vi "ClientTake2.vi"() -> ()   [LabVIEW 2021]
panel:
  in  "stop":bool
  in  "C6":bool
  in  "C5":bool
  in  "C4":bool
  in  "C3":bool
  in  "C2":bool
  in  "C1":bool
  in  "B6":bool
  in  "B5":bool
  in  "B4":bool
  in  "B3":bool
  in  "B2":bool
  in  "B1":bool
  in  "A6":bool
  in  "A5":bool
  in  "A4":bool
  in  "A3":bool
  in  "A2":bool
  in  "A1":bool
  # "1"
  # "2"
  # "3"
  # "4"
  # "5"
  # "6"
  # "Alarm Switches"
  # "Zone"
  # "Bypass Switches"
  # "Tamper Switches"
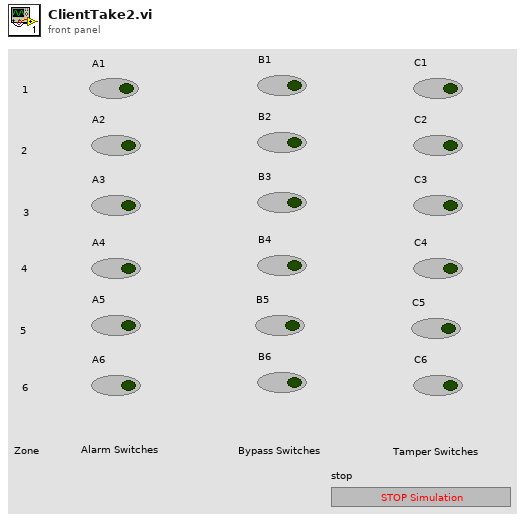
[diagram p1: front panel]
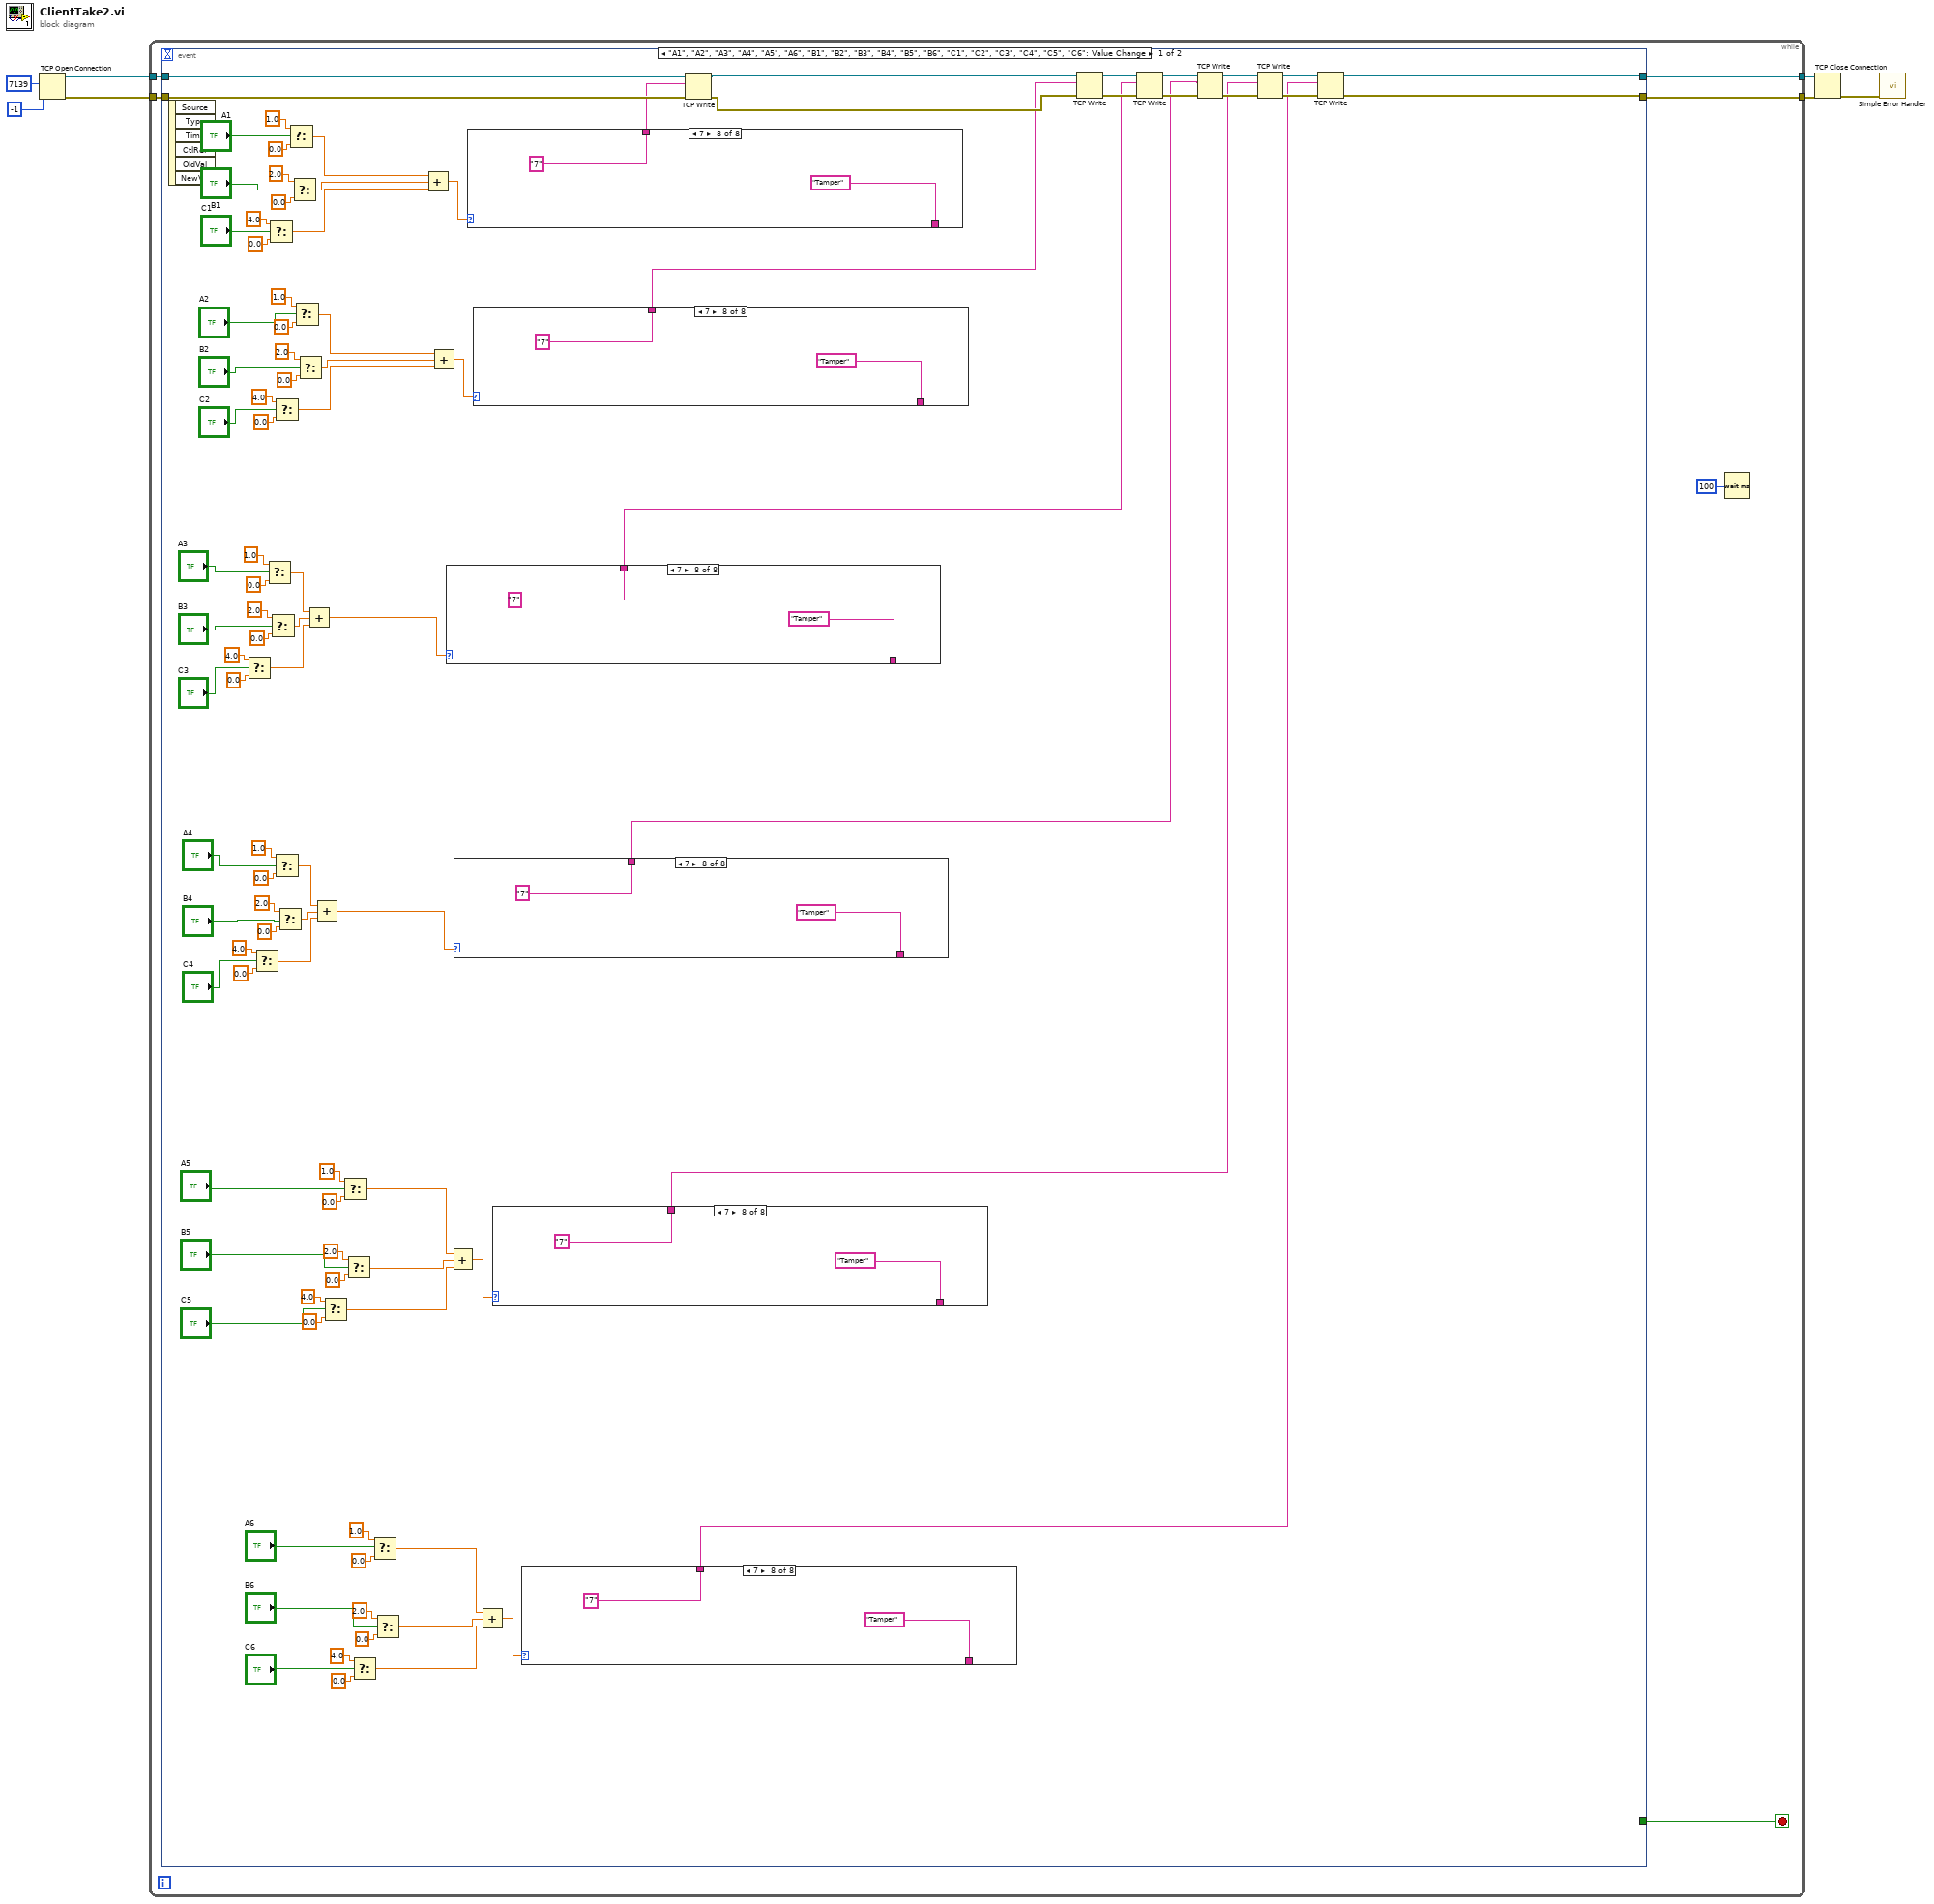
[diagram p0: block diagram]
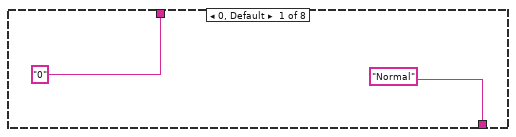
[diagram p2: hidden frame]
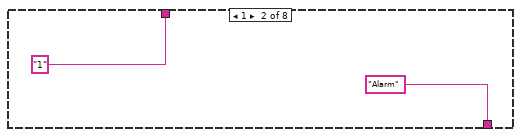
[diagram p3: hidden frame]
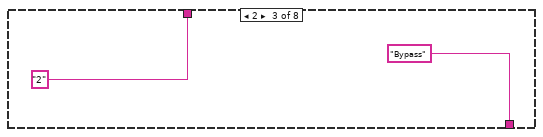
[diagram p4: hidden frame]
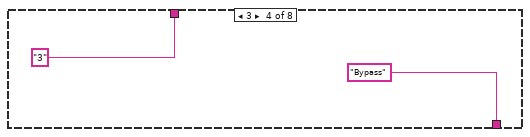
[diagram p5: hidden frame]
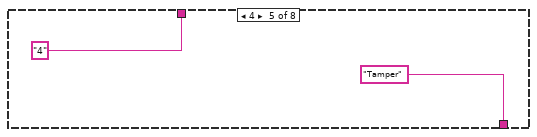
[diagram p6: hidden frame]
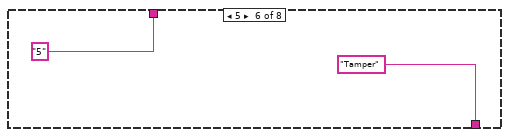
[diagram p7: hidden frame]
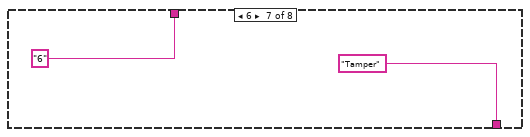
[diagram p8: hidden frame]
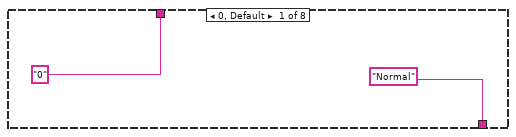
[diagram p9: hidden frame]
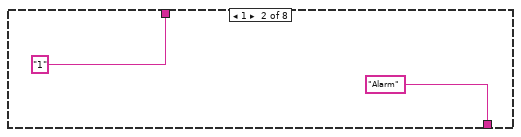
[diagram p10: hidden frame]
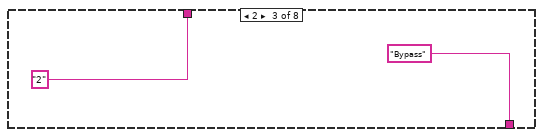
[diagram p11: hidden frame]
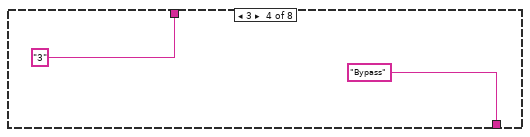
[diagram p12: hidden frame]
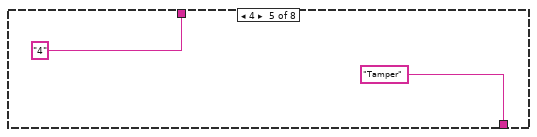
[diagram p13: hidden frame]
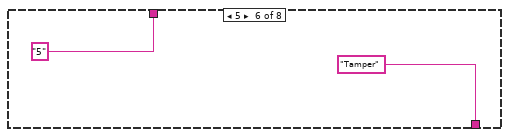
[diagram p14: hidden frame]
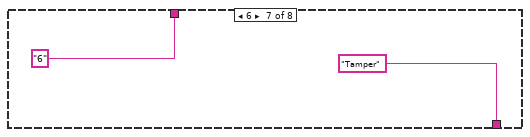
[diagram p15: hidden frame]
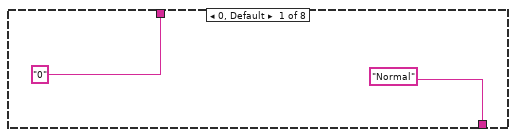
[diagram p16: hidden frame]
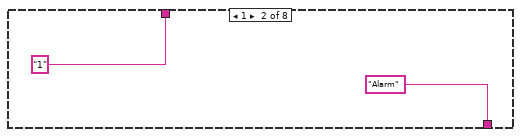
[diagram p17: hidden frame]
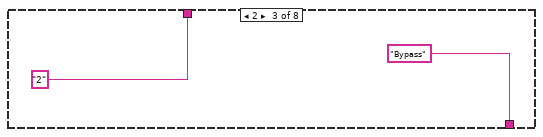
[diagram p18: hidden frame]
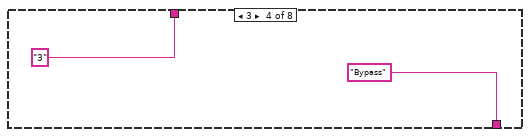
[diagram p19: hidden frame]
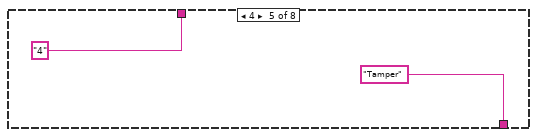
[diagram p20: hidden frame]
diagram:
  n1 = TCP Open Connection(remote port or service name=u16 7139, timeout ms (60000)=-1) -> (connection ID=w7:refnum<k5>, error out=w5:errorcluster)  [unwired: 3 in]
  n2 = while {
    tunnel: w7 -> [w13]
    tunnel: [w10] -> w6
    tunnel: w5 -> [w12]
    tunnel: [w9] -> w4
    stop <- w8 stop-if-true
    n3 = event shown="[0] \"A1\", \"A2\", \"A3\", \"A4\", \"A5\", \"A6\", \"B1\", \"B2\", \"B3\", \"B4\", \"B5\", \"B6\", \"C1\", \"C2\", \"C3\", \"C4\", \"C5\", \"C6\": Value Change" {
      selector: _ -> [_ _]
      dyn-events: _ -> [_ _]
      timeout: _ -> [_ _]
      tunnel: w13 -> [w99 _]
      tunnel: w12 -> [w98 _]
      tunnel: [w61 _] -> w10
      tunnel: [w66 _] -> w9
      tunnel: [_ "stop"] -> w8
      event "A1", "A2", "A3", "A4", "A5", "A6", "B1", "B2", "B3", "B4", "B5", "B6", "C1", "C2", "C3", "C4", "C5", "C6": Value Change {
        n4 = event-data() -> ()  [unwired: 1 in, 6 out]
        n5 = Select(t=4.0, s="C3", f=0.0) -> (s? t:f=w73:dbl)
        n6 = Select(t=4.0, s="C4", f=0.0) -> (s? t:f=w52:dbl)
        n7 = Select(t=1.0, s="A3", f=0.0) -> (s? t:f=w78:dbl)
        n8 = Select(t=4.0, s="C1", f=0.0) -> (s? t:f=w102:dbl)
        n9 = Select(t=2.0, s="B3", f=0.0) -> (s? t:f=w74:dbl)
        n10 = Select(t=4.0, s="C2", f=0.0) -> (s? t:f=w89:dbl)
        n11 = Select(t=1.0, s="A4", f=0.0) -> (s? t:f=w57:dbl)
        n12 = Select(t=2.0, s="B4", f=0.0) -> (s? t:f=w53:dbl)
        n13 = Select(t=1.0, s="A1", f=0.0) -> (s? t:f=w108:dbl)
        n14 = Select(t=2.0, s="B1", f=0.0) -> (s? t:f=w103:dbl)
        n15 = Select(t=1.0, s="A2", f=0.0) -> (s? t:f=w94:dbl)
        n16 = Select(t=2.0, s="B2", f=0.0) -> (s? t:f=w90:dbl)
        n17 = Compound Arithmetic op=ADD(w78, w74, w73) -> (w71:dbl)
        n18 = Compound Arithmetic op=ADD(w57, w53, w52) -> (w50:dbl)
        n19 = Select(t=4.0, s="C5", f=0.0) -> (s? t:f=w22:dbl)
        n20 = Select(t=1.0, s="A5", f=0.0) -> (s? t:f=w27:dbl)
        n21 = Select(t=2.0, s="B5", f=0.0) -> (s? t:f=w23:dbl)
        n22 = Select(t=4.0, s="C6", f=0.0) -> (s? t:f=w42:dbl)
        n23 = Select(t=1.0, s="A6", f=0.0) -> (s? t:f=w47:dbl)
        n24 = Select(t=2.0, s="B6", f=0.0) -> (s? t:f=w43:dbl)
        n25 = Compound Arithmetic op=ADD(w108, w103, w102) -> (w81:dbl)
        n26 = Compound Arithmetic op=ADD(w94, w90, w89) -> (w14:dbl)
        n27 = case shown="7" w71 {
          tunnel: ["0" "1" "2" "3" "4" "5" "6" "7"] -> w60
          tunnel: ["Normal" "Alarm" "Bypass" "Bypass" "Tamper" "Tamper" "Tamper" "Tamper"] -> _
          frame 0, Default {
          }
          frame 1 {
          }
          frame 2 {
          }
          frame 3 {
          }
          frame 4 {
          }
          frame 5 {
          }
          frame 6 {
          }
          frame 7 {
          }
        }
        n28 = case shown="7" w50 {
          tunnel: ["0" "1" "2" "3" "4" "5" "6" "7"] -> w33
          tunnel: ["Normal" "Alarm" "Bypass" "Bypass" "Tamper" "Tamper" "Tamper" "Tamper"] -> _
          frame 0, Default {
          }
          frame 1 {
          }
          frame 2 {
          }
          frame 3 {
          }
          frame 4 {
          }
          frame 5 {
          }
          frame 6 {
          }
          frame 7 {
          }
        }
        n29 = Compound Arithmetic op=ADD(w27, w23, w22) -> (w20:dbl)
        n30 = case shown="7" w81 {
          tunnel: ["0" "1" "2" "3" "4" "5" "6" "7"] -> w97
          tunnel: ["Normal" "Alarm" "Bypass" "Bypass" "Tamper" "Tamper" "Tamper" "Tamper"] -> _
          frame 0, Default {
          }
          frame 1 {
          }
          frame 2 {
          }
          frame 3 {
          }
          frame 4 {
          }
          frame 5 {
          }
          frame 6 {
          }
          frame 7 {
          }
        }
        n31 = case shown="7" w14 {
          tunnel: ["0" "1" "2" "3" "4" "5" "6" "7"] -> w82
          tunnel: ["Normal" "Alarm" "Bypass" "Bypass" "Tamper" "Tamper" "Tamper" "Tamper"] -> _
          frame 0, Default {
          }
          frame 1 {
          }
          frame 2 {
          }
          frame 3 {
          }
          frame 4 {
          }
          frame 5 {
          }
          frame 6 {
          }
          frame 7 {
          }
        }
        n32 = Compound Arithmetic op=ADD(w47, w43, w42) -> (w40:dbl)
        n33 = case shown="7" w20 {
          tunnel: ["0" "1" "2" "3" "4" "5" "6" "7"] -> w16
          tunnel: ["Normal" "Alarm" "Bypass" "Bypass" "Tamper" "Tamper" "Tamper" "Tamper"] -> _
          frame 0, Default {
          }
          frame 1 {
          }
          frame 2 {
          }
          frame 3 {
          }
          frame 4 {
          }
          frame 5 {
          }
          frame 6 {
          }
          frame 7 {
          }
        }
        n34 = case shown="7" w40 {
          tunnel: ["0" "1" "2" "3" "4" "5" "6" "7"] -> w15
          tunnel: ["Normal" "Alarm" "Bypass" "Bypass" "Tamper" "Tamper" "Tamper" "Tamper"] -> _
          frame 0, Default {
          }
          frame 1 {
          }
          frame 2 {
          }
          frame 3 {
          }
          frame 4 {
          }
          frame 5 {
          }
          frame 6 {
          }
          frame 7 {
          }
        }
        n35 = TCP Write(connection ID=w99, data in=w97, error in (no error)=w98) -> (connection ID out=w84:refnum<k5>, error out=w83:errorcluster)  [unwired: 1 in, 1 out]
        n36 = TCP Write(connection ID=w84, data in=w82, error in (no error)=w83) -> (connection ID out=w65:refnum<k5>, error out=w70:errorcluster)  [unwired: 1 in, 1 out]
        n37 = TCP Write(connection ID=w65, data in=w60, error in (no error)=w70) -> (connection ID out=w64:refnum<k5>, error out=w69:errorcluster)  [unwired: 1 in, 1 out]
        n38 = TCP Write(connection ID=w64, data in=w33, error in (no error)=w69) -> (connection ID out=w63:refnum<k5>, error out=w68:errorcluster)  [unwired: 1 in, 1 out]
        n39 = TCP Write(connection ID=w63, data in=w16, error in (no error)=w68) -> (connection ID out=w62:refnum<k5>, error out=w67:errorcluster)  [unwired: 1 in, 1 out]
        n40 = TCP Write(connection ID=w62, data in=w15, error in (no error)=w67) -> (connection ID out=w61:refnum<k5>, error out=w66:errorcluster)  [unwired: 1 in, 1 out]
      }
      event "stop": Value Change {
        n41 = event-data() -> ()  [unwired: 1 in, 6 out]
      }
    }
    n42 = Wait (ms)(milliseconds to wait=u32 100) -> ()  [unwired: 1 out]
  }
  n43 = TCP Close Connection(connection ID=w6, error in (no error)=w4) -> (error out=w1:errorcluster)  [unwired: 1 in, 1 out]
  n44 = call <vilib>:"Simple Error Handler.vi"("error in (no error)"=w1) -> ()  [unwired: 4 in, 5 out]
